vi "open camera.vi"(8 "error in (no error)":errorcluster, 9 "Camera Settings":path, 10 "serial number":string, 11 "driver":T2) -> (0 "error out":errorcluster, 2 "Camera":T1)   [LabVIEW 2022 SP3, in "Vision.lvlib"]
uses:
  Vision.lvlib
  camera driver.ctl
  camera.ctl
  C:/Users/Caleb/Desktop/nebraska-silicon-lab/pixel-gantry-control/Gantry/Shared Components/External/bin/uEyeDotNet.dll
  bin/uEyeDotNet.dll
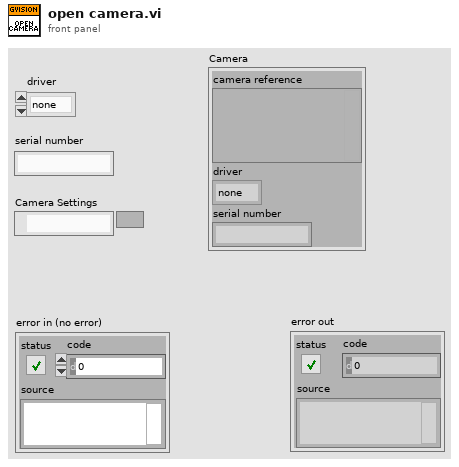
[diagram p1: front panel]
types:
  T1 = typedef "Vision.lvlib/camera.ctl" = cluster{"camera reference":variant, "driver":T2, "serial number":string}
  T2 = typedef "Vision.lvlib/camera driver.ctl" = enum16{"none", "ueye"}
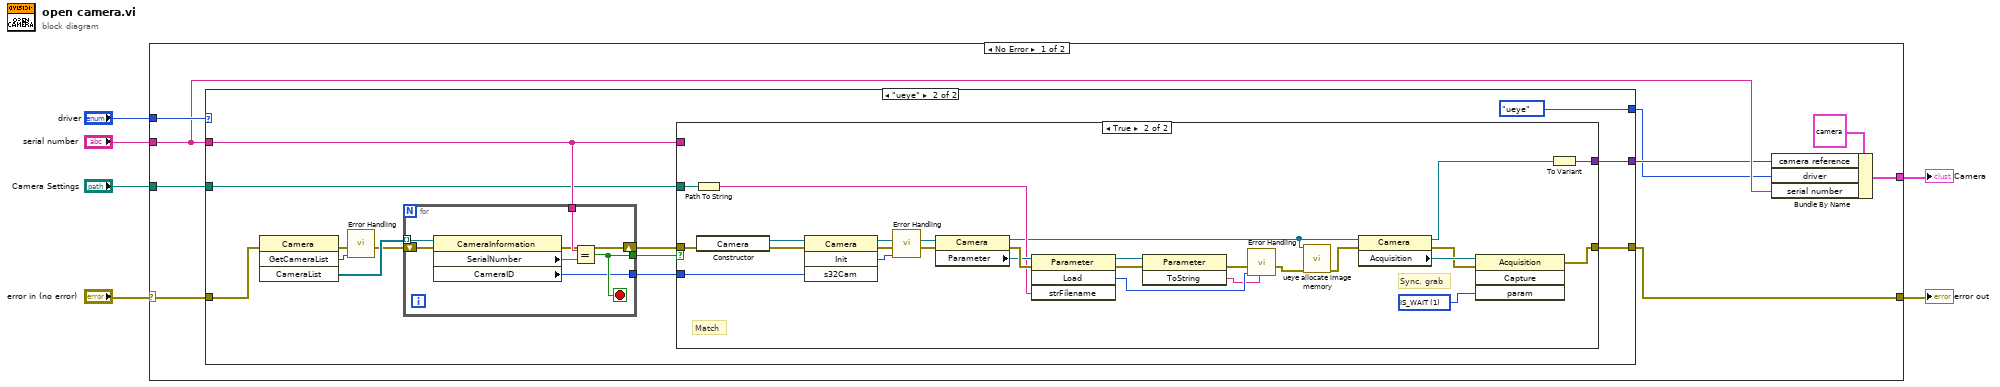
[diagram p0: block diagram]
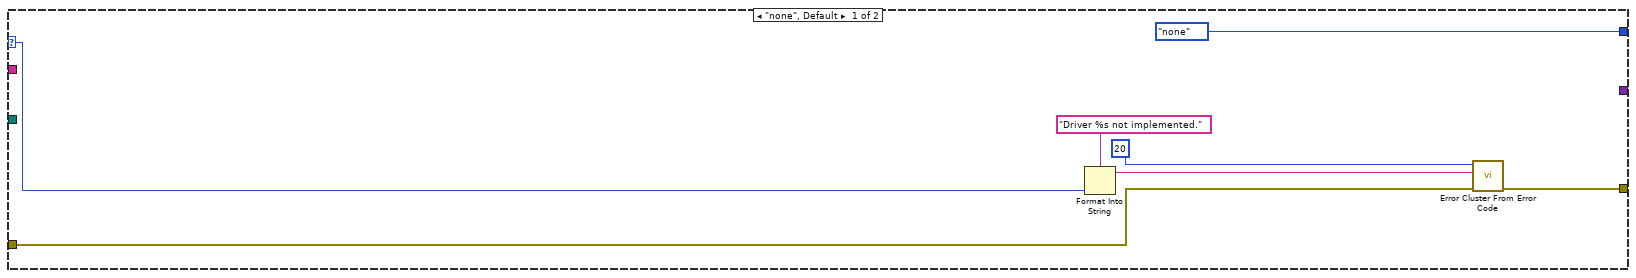
[diagram p2: hidden frame]
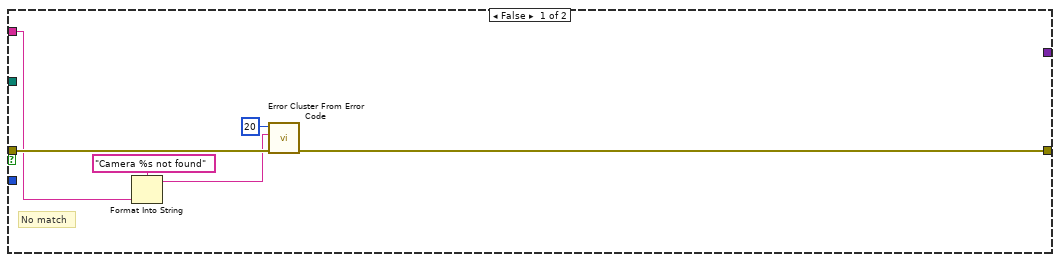
[diagram p3: hidden frame]
diagram:
  n1 = case shown="No Error" "error in (no error)" {
    selector: "error in (no error)" -> [w14 w75]
    tunnel: [w8 w75] -> w5
    tunnel: "driver" -> [w11 _]
    tunnel: "serial number" -> [w10 _]
    tunnel: "Camera Settings" -> [w15 _]
    tunnel: [w12 _] -> w1
    frame No Error {
      n2 = case shown="\"ueye\"" w11 {
        selector: w11 -> [w18 _]
        tunnel: w10 -> [_ w27]
        tunnel: w15 -> [_ w23]
        tunnel: w14 -> [w21 w35]
        tunnel: [_ w26] -> w9
        tunnel: [w20 w25] -> w8
        tunnel: [camera_driver."none" ("driver") camera_driver."ueye" ("driver")] -> w7
        frame "none", Default {
          n3 = Format Into String(format string="Driver %s not implemented.", w18) -> (resulting string=w17:string)  [unwired: 2 in, 1 out]
          n4 = call <vilib>:"Error Cluster From Error Code.vi"("error in (no error)"=w21, "error message (\"\")"=w17, "error code (0)"=20) -> ("error out"=w20:errorcluster)  [unwired: 6 in]
        }
        frame "ueye" {
          n5 = invoke on="Methodenknoten" class="Camera" method="GetCameraList"(error in=w35) -> (error out=w30:errorcluster, "GetCameraList"=w29:i32, "CameraList"=w34:refnum<k24>[])  [unwired: 3 in, 1 out]
          n6 = call "Error Handling.vi"("Error Code"=w29, "Error In"=w30) -> ("Error Out"=w28:errorcluster)  [unwired: 9 in]
          n7 = for {
            tunnel: w34 -> [w74] mode=indexing
            tunnel: w27 -> [w73]
            tunnel: [w71] -> w33
            shift-right: [w69] -> w32
            shift-left: w28 -> [w70]
            tunnel: [w68] -> w31
            stop <- w71 stop-if-true
            n8 = property class="CameraInformation"(reference=w74, error in=w70) -> (error out=w69:errorcluster, "SerialNumber"=w72:string, "CameraID"=w68:i64)  [unwired: 1 out]
            n9 = Equal?(x=w73, y=w72) -> (x = y?=w71:bool)
          }
          n10 = case shown="True" w33 {
            tunnel: w32 -> [w41 w67]
            tunnel: w31 -> [_ w65]
            tunnel: [w40 w45] -> w25
            tunnel: w27 -> [w37 _]
            tunnel: [_ w59] -> w26
            tunnel: w23 -> [_ w51]
            frame False {
              # "No match"
              n11 = Format Into String(format string="Camera %s not found" ("error message (\"\")"), w37) -> (resulting string=w36:string)  [unwired: 2 in, 1 out]
              n12 = call <vilib>:"Error Cluster From Error Code.vi"("error in (no error)"=w41, "error message (\"\")"=w36, "error code (0)"=20) -> ("error out"=w40:errorcluster)  [unwired: 6 in]
            }
            frame True {
              w60 = 1 items=["IS_DONT_WAIT", "IS_WAIT"] ("Wait")
              # "Sync. grab"
              # "Match"
              n13 = Path To String(path=w51) -> (string=w50:string)
              n14 = constructor class="Camera"(error in=w67) -> (reference out=w49:refnum<k24>, error out=w66:errorcluster)  [unwired: 2 in, 1 out]
              n15 = invoke class="Camera" method="Init"(reference=w49, error in=w66, "s32Cam"=w65) -> (reference out=w48:refnum<k24>, error out=w64:errorcluster, "Init"=w63:i32)  [unwired: 1 in, 1 out]
              n16 = call "Error Handling.vi"("Error Code"=w63, "Error In"=w64) -> ("Error Out"=w47:errorcluster)  [unwired: 9 in]
              n17 = property class="Camera"(reference=w48, error in=w47) -> (reference out=w42:refnum<k24>, error out=w56:errorcluster, "Parameter"=w55:refnum<k24>)
              n18 = invoke class="Parameter" method="Load"(reference=w55, error in=w56, "strFilename"=w50) -> (reference out=w57:refnum<k24>, error out=w58:errorcluster, "Load"=w54:i32)  [unwired: 1 in, 1 out]
              n19 = invoke class="Parameter" method="ToString"(reference=w57, error in=w58) -> (error out=w53:errorcluster, "ToString"=w52:string)  [unwired: 1 in, 1 out]
              n20 = call "Error Handling.vi"("Error String"=w52, "Error Code"=w54, "Error In"=w53) -> ("Error Out"=w44:errorcluster)  [unwired: 8 in]
              n21 = call "ueye allocate image memory.vi"(".NET (Reference)"=w42, "Error In"=w44) -> ("Error Out"=w43:errorcluster)  [unwired: 13 in, 4 out]
              n22 = property class="Camera"(reference=w42, error in=w43) -> (reference out=w46:refnum<k24>, error out=w61:errorcluster, "Acquisition"=w62:refnum<k24>)
              n23 = invoke class="Acquisition" method="Capture"(reference=w62, error in=w61, "param"=w60) -> (error out=w45:errorcluster)  [unwired: 1 in, 3 out]
              n24 = To Variant(anything=w46) -> (Variant=w59:variant)
            }
          }
        }
      }
      n25 = Bundle By Name(cluster=T1 {"camera reference"=variant, "driver"=enum."none", "serial number"=""}, "camera reference"=w9, "driver"=w7, "serial number"=w10) -> (w12:T1)
    }
    frame Error {
    }
  }
  "error out" <- w5
  "Camera" <- w1
